vi "Calibration INI File.vi"   [LabVIEW 2011]
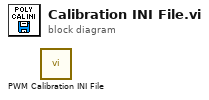
[diagram p0: block diagram]
diagram:
  n1 = call "PWM Calibration INI File.vi"() -> ()  [unwired: 10 in, 2 out]
